vi "Write Scan start.vi"(8 "error in (no error)":errorcluster, 10 "Scan start":timestamp, 11 "Mapping params in":refnum<class "CV-Mapping.lvclass">) -> (0 "error out":errorcluster, 3 "Mapping params out":refnum<class "CV-Mapping.lvclass">)   [LabVIEW 2013, in "CameraVision.lvlib" / "CV-Mapping.lvclass"]
uses:
  CV-Mapping.lvclass
  CV-Mapping.lvclass/CV-Mapping.ctl
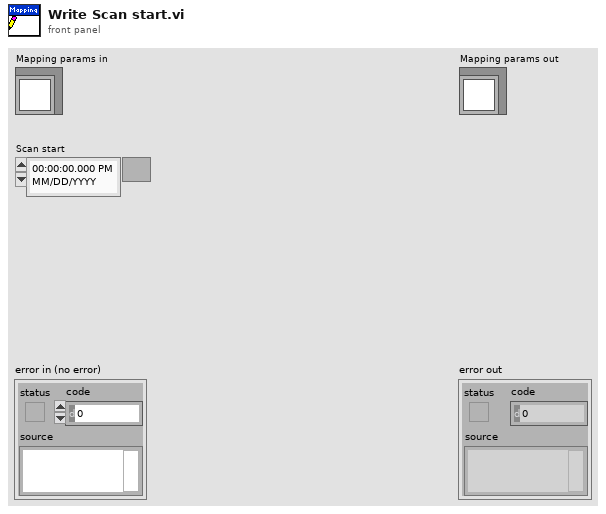
[diagram p1: front panel]
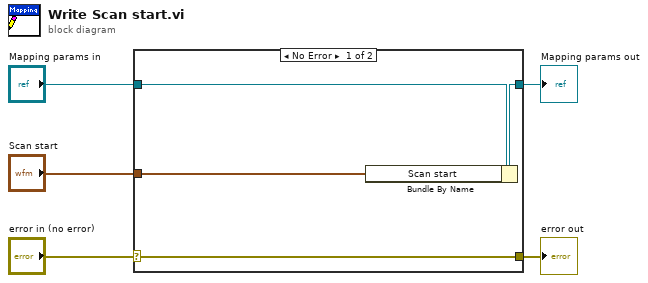
[diagram p0: block diagram]
diagram:
  n1 = case shown="No Error" "error in (no error)" {
    selector: "error in (no error)" -> [w9 w10]
    tunnel: [w9 w10] -> w4
    tunnel: [w7 w11] -> w2
    tunnel: "Mapping params in" -> [w8 w11]
    tunnel: "Scan start" -> [w6 _]
    frame No Error {
      n2 = Bundle By Name(cluster=w8, "Scan start"=w6) -> (w7:refnum<class "CV-Mapping.lvclass">)
    }
    frame Error {
    }
  }
  "error out" <- w4
  "Mapping params out" <- w2
